vi "Binary Config With Single Term Class Unit Tests.vi"(8 "error in (no error)":errorcluster) -> (0 "error out":errorcluster)   [LabVIEW 2021]
uses:
  Source/Abs_Types/Boolean/Abs_Boolean.lvclass
  C:/New folder/LV_Abstract/LV_Abstract/Source/Abs_Types/Type/Abs_Type.lvclass
  Source/Abs_Types/Double Float/Abs_Double Float.lvclass
  Source/Abs_Types/Extended Float/Abs_Extended Float.lvclass
  Source/Abs_Types/Single Float/Abs_Single Float.lvclass
  Source/Abs_Types/Time/Abs_Time.lvclass
  Source/Abs_Types/Complex Double Float/Abs_Complex Double Float.lvclass
  Source/Abs_Types/Complex Extended Float/Abs_Complex Extended Float.lvclass
  Source/Abs_Types/Complex Single Float/Abs_Complex Single Float.lvclass
  Source/Abs_Types/I8 Integer/Abs_I8 Integer.lvclass
  Source/Abs_Types/I16 Integer/Abs_I16 Integer.lvclass
  Source/Abs_Types/I32 Integer/Abs_I32 Integer.lvclass
  Source/Abs_Types/I64 Integer/Abs_I64 Integer.lvclass
  Source/Abs_Types/U8 Integer/Abs_U8 Integer.lvclass
  Source/Abs_Types/U16 Integer/Abs_U16 Integer.lvclass
  Source/Abs_Types/U32 Integer/Abs_U32 Integer.lvclass
  Source/Abs_Types/U64 Integer/Abs_U64 Integer.lvclass
  Source/Abs_Types/String/Abs_String.lvclass
  ec70d7ea-8a3d-4754-ba28-d4fe5c722101.vi
  b6c2acd6-c644-432a-9b1c-c9fcc0820943.vi
  30c2e6e1-3486-4832-8975-47388ff2611a.vi
  a5d5bd5a-def4-49ba-bdc0-524ad19b816e.vi
  1110239c-6e8d-45dc-a6ef-38f97f16d6c8.vi
  dfda7940-254e-4b81-9033-01cea9b2eb8b.vi
  29149eef-2b65-4fa7-b0fd-00a2aba6bb2a.vi
  0af03642-7583-44ad-a16d-f5ef4bedefd9.vi
  8d20b177-a927-4a2f-b4ed-51e929c5ec88.vi
  228df6da-9157-4bdf-8598-ce3ac85fe975.vi
  6ef478d1-abc9-4543-9bfd-3817465b62e1.vi
  957f6fde-f444-47e3-a0ca-c16bc0ee107e.vi
  990241af-0d33-409b-9b41-12d506eae33b.vi
  069cd166-5e64-46e3-ab3e-142203c796d9.vi
  e1cfd4a5-c225-47c4-bcd4-e8422310f8ac.vi
  07454bd2-52aa-46e8-9371-7bd7db9b227a.vi
  126b08aa-30fa-44da-a4ab-573a30548618.vi
  Source/Abs_Types/Abs_Simple_Read.vi
  Source/Abs_Types/Boolean/Simple Read.vi
  Source/Abs_Types/String/Simple Read.vi
  Source/Abs_Types/Time/Simple Read.vi
  Source/Abs_Types/Double Float/Simple Read.vi
  Source/Abs_Types/Extended Float/Simple Read.vi
  Source/Abs_Types/Single Float/Simple Read.vi
  Source/Abs_Types/I8 Integer/Simple Read.vi
  Source/Abs_Types/I16 Integer/Simple Read.vi
  Source/Abs_Types/I32 Integer/Simple Read.vi
  Source/Abs_Types/I64 Integer/Simple Read.vi
  Source/Abs_Types/U8 Integer/Simple Read.vi
  Source/Abs_Types/U16 Integer/Simple Read.vi
  Source/Abs_Types/U32 Integer/Simple Read.vi
  Source/Abs_Types/U64 Integer/Simple Read.vi
  Source/Constants/Support/Time/Const_Time.lvclass
  C:/New folder/LV_Abstract/LV_Abstract/Source/Abs_Types/Time/Abs_Time.lvclass
  <vilib>/Utility/Data Type/Get Type Information.vi
  Source/Constants/Abs_Constant.vi
  Source/Constants/Support/Bool/Bool.vi
  Source/Functions/Logic/NOT.vi
  Source/Functions/Logic/Support/NOT/Bool/Method.vi
  <vilib>/addons/_JKI Toolkits/Caraya/classes/Test/Define Test.vi
  Source/Abs_Types/Type/Read Config Binary.vi
  <vilib>/addons/_JKI Toolkits/Caraya/classes/Assert/Assert.vi
  <vilib>/addons/_JKI Toolkits/Caraya/classes/Assert/Assert Equal Value_Variant.vi
  <vilib>/addons/_JKI Toolkits/Caraya/classes/Assert/Assert Equal Type_Variant.vi
  Source/Constants/Support/Str/Str.vi
  Source/Constants/Support/Time/Time.vi
  Source/Functions/Math/Increment.vi
  Source/Functions/Math/Support/Increment/Time/Method.vi
  Source/Constants/Support/DBL/DBL.vi
  Source/Constants/Support/EXT/EXT.vi
  Source/Constants/Support/SGL/SGL.vi
  Source/Constants/Support/CPLX_DBL/CPLX_DBL.vi
  Source/Abs_Types/Complex Double Float/Simple Read.vi
  Source/Constants/Support/CPLX_EXT/CPLX_EXT.vi
  Source/Abs_Types/Complex Extended Float/Simple Read.vi
  Source/Constants/Support/CPLX_SGL/CPLX_SGL.vi
  Source/Abs_Types/Complex Single Float/Simple Read.vi
  Source/Constants/Support/I8/I8.vi
  Source/Constants/Support/I16/I16.vi
  Source/Constants/Support/I32/I32.vi
  Source/Constants/Support/I64/I64.vi
  Source/Constants/Support/U8/U8.vi
  Source/Constants/Support/U16/U16.vi
  Source/Constants/Support/U32/U32.vi
  Source/Constants/Support/U64/U64.vi
  Source/Constants/Support/DBL/Const_DBL.lvclass
  Source/Constants/Support/U8/Const_U8.lvclass
  Source/Constants/Support/U16/Const_U16.lvclass
  Source/Constants/Support/U32/Const_U32.lvclass
  Source/Constants/Support/U64/Const_U64.lvclass
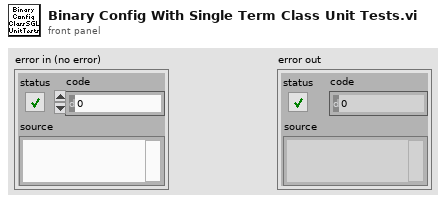
[diagram p1: front panel]
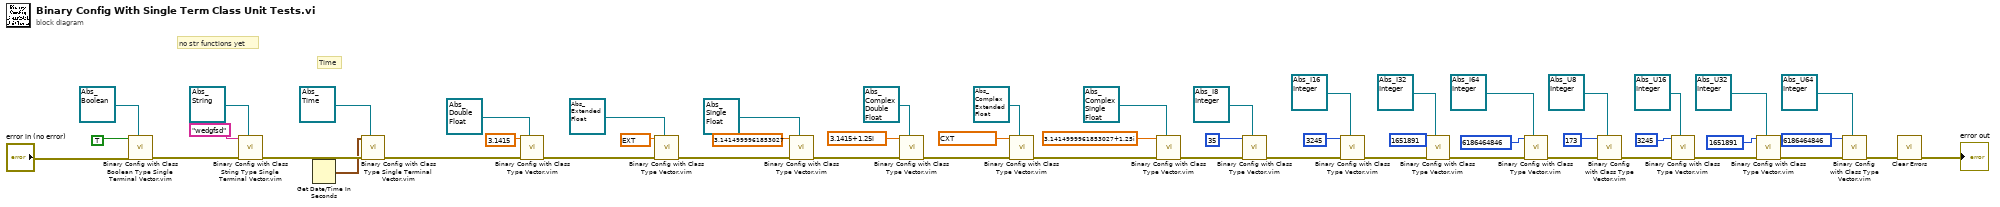
[diagram p0: block diagram]
diagram:
  # "no str functions yet"
  # "Time"
  n1 = call "Binary Config with Class Boolean Type Single Terminal Vector.vim"("Expected Class"=refnum<class "Abs_Boolean.lvclass"> refnum ("Abs_Boolean.lvclass"), "error in (no error)"="error in (no error)", "Test Value"=TRUE) -> ("error out"=w43:errorcluster)  [unwired: 8 in]
  n2 = call "Binary Config with Class String Type Single Terminal Vector.vim"("Expected Class"=refnum<class "Abs_String.lvclass"> refnum ("Abs_String.lvclass"), "error in (no error)"=w43, "Test Value"="wedgfsd") -> ("error out"=w42:errorcluster)  [unwired: 8 in]
  n3 = Get Date/Time In Seconds() -> (seconds since 1Jan1904=w39:timestamp)
  n4 = call "Binary Config with Class Type Single Terminal Vector.vim"("Abs_Double Float.lvclass"=refnum<class "Abs_Time.lvclass"> refnum ("Abs_Time.lvclass"), "error in (no error)"=w42, "Test Value"=w39) -> ("error out"=w41:errorcluster)  [unwired: 8 in]
  n5 = call "Binary Config with Class Type Vector.vim"("Expected Class"=refnum<class "Abs_Double Float.lvclass"> refnum ("Class"), "error in (no error)"=w41, "Test Value"=3.1415) -> ("error out"=w49:errorcluster)  [unwired: 8 in]
  n6 = call "Binary Config with Class Type Vector.vim"("Expected Class"=refnum<class "Abs_Extended Float.lvclass"> refnum ("Abs_Extended Float.lvclass"), "error in (no error)"=w49, "Test Value"=ext 3.1414999999999999999) -> ("error out"=w45:errorcluster)  [unwired: 8 in]
  n7 = call "Binary Config with Class Type Vector.vim"("Expected Class"=refnum<class "Abs_Single Float.lvclass"> refnum ("Abs_Single Float.lvclass"), "error in (no error)"=w45, "Test Value"=sgl 3.1415) -> ("error out"=w37:errorcluster)  [unwired: 8 in]
  n8 = call "Binary Config with Class Type Vector.vim"("Expected Class"=refnum<class "Abs_Complex Double Float.lvclass"> refnum ("Abs_Complex Double Float.lvclass"), "error in (no error)"=w37, "Test Value"=cdb 3.1415+1.25i) -> ("error out"=w34:errorcluster)  [unwired: 8 in]
  n9 = call "Binary Config with Class Type Vector.vim"("Expected Class"=refnum<class "Abs_Complex Extended Float.lvclass"> refnum ("Abs_Complex Extended Float.lvclass"), "error in (no error)"=w34, "Test Value"=cxt 3.1415+1.25i) -> ("error out"=w31:errorcluster)  [unwired: 8 in]
  n10 = call "Binary Config with Class Type Vector.vim"("Expected Class"=refnum<class "Abs_Complex Single Float.lvclass"> refnum ("Abs_Complex Single Float.lvclass"), "error in (no error)"=w31, "Test Value"=csg 3.1415+1.25i) -> ("error out"=w29:errorcluster)  [unwired: 8 in]
  n11 = call "Binary Config with Class Type Vector.vim"("Expected Class"=refnum<class "Abs_I8 Integer.lvclass"> refnum ("Abs_I8 Integer.lvclass"), "error in (no error)"=w29, "Test Value"=i8 35) -> ("error out"=w25:errorcluster)  [unwired: 8 in]
  n12 = call "Binary Config with Class Type Vector.vim"("Expected Class"=refnum<class "Abs_I16 Integer.lvclass"> refnum ("Abs_I16 Integer.lvclass"), "error in (no error)"=w25, "Test Value"=i16 3245) -> ("error out"=w22:errorcluster)  [unwired: 8 in]
  n13 = call "Binary Config with Class Type Vector.vim"("Expected Class"=refnum<class "Abs_I32 Integer.lvclass"> refnum ("Abs_I32 Integer.lvclass"), "error in (no error)"=w22, "Test Value"=1651891) -> ("error out"=w19:errorcluster)  [unwired: 8 in]
  n14 = call "Binary Config with Class Type Vector.vim"("Expected Class"=refnum<class "Abs_I64 Integer.lvclass"> refnum ("Abs_I64 Integer.lvclass"), "error in (no error)"=w19, "Test Value"=i64 6186464846) -> ("error out"=w16:errorcluster)  [unwired: 8 in]
  n15 = call "Binary Config with Class Type Vector.vim"("Expected Class"=refnum<class "Abs_U8 Integer.lvclass"> refnum ("Abs_U8 Integer.lvclass"), "error in (no error)"=w16, "Test Value"=u8 173) -> ("error out"=w14:errorcluster)  [unwired: 8 in]
  n16 = call "Binary Config with Class Type Vector.vim"("Expected Class"=refnum<class "Abs_U16 Integer.lvclass"> refnum ("Abs_U16 Integer.lvclass"), "error in (no error)"=w14, "Test Value"=u16 3245) -> ("error out"=w11:errorcluster)  [unwired: 8 in]
  n17 = call "Binary Config with Class Type Vector.vim"("Expected Class"=refnum<class "Abs_U32 Integer.lvclass"> refnum ("Abs_U32 Integer.lvclass"), "error in (no error)"=w11, "Test Value"=u32 1651891) -> ("error out"=w8:errorcluster)  [unwired: 8 in]
  n18 = call "Binary Config with Class Type Vector.vim"("Expected Class"=refnum<class "Abs_U64 Integer.lvclass"> refnum ("Abs_U64 Integer.lvclass"), "error in (no error)"=w8, "Test Value"=u64 6186464846) -> ("error out"=w5:errorcluster)  [unwired: 8 in]
  n19 = call <vilib>:"Clear Errors.vi"("error in (no error)"=w5) -> ("error out"=→"error out":errorcluster)  [unwired: 5 in, 1 out]
